vi "FindMessageSet.vi"(11 "ConcreteActor.lvclass":variant) -> (3 "MessageSet":T1)   [LabVIEW 2020, in "jettl.lvlib"]
uses:
  jettl.lvlib
  Message/Message.lvclass
  MessageSet.ctl
  <vilib>/Utility/Data Type/NI_Data Type.lvlib
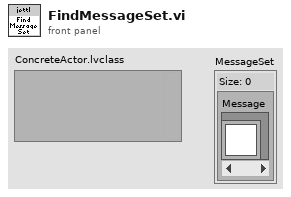
[diagram p1: front panel]
types:
  T1 = typedef "jettl.lvlib/MessageSet.ctl" = set{refnum<class "Message.lvclass">}
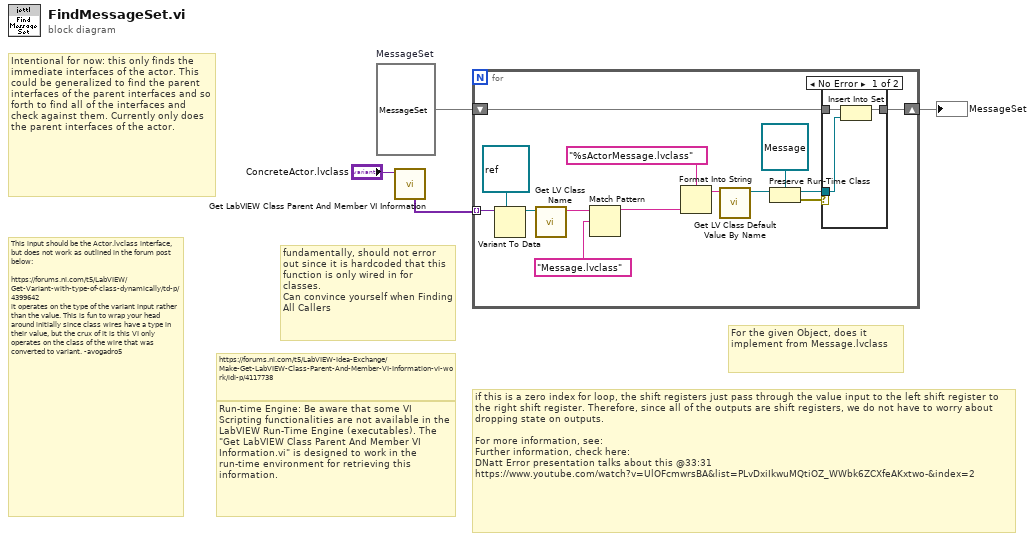
[diagram p0: block diagram]
diagram:
  w4 = T1 {}  # MessageSet
  # "fundamentally, should not error out since it is hardcoded that this function is only wired in for classes.\nCan convince yourself when Finding All Callers"
  # "if this is a zero index for loop, the shift registers just pass through the value input to the left shift register to the right shift register. Therefore, since all of the outputs are shift registers, we do not have to worry about dropping state on outputs.\n\nFor more information, see:\nFurther information, check here:\nDNatt Error presentation talks about this @33:31\nhttps://www.youtube.com/watch?v=UlOFcmwrsBA&list=PLvDxiIkwuMQtiOZ_WWbk6ZCXfeAKxtwo-&index=2"
  # "For the given Object, does it implement from Message.lvclass"
  # "This input should be the Actor.lvclass interface, but does not work as outlined in the forum post below:\n\nhttps://forums.ni.com/t5/LabVIEW/Get-Variant-with-type-of-class-dynamically/td-p/4399642\nit operates on the type of the variant input rather than the value. This is fun to wrap your head around initially since class wires have a type in their value, but the crux of it is this VI only operates on the class of the wire that was converted to variant. -avogadro5"
  # "Intentional for now: this only finds the immediate interfaces of the actor. This could be generalized to find the parent interfaces of the parent interfaces and so forth to find all of the interfaces and check against them. Currently only does the parent interfaces of the actor."
  # "Run-time Engine: Be aware that some VI Scripting functionalities are not available in the LabVIEW Run-Time Engine (executables). The \"Get LabVIEW Class Parent And Member VI Information.vi\" is designed to work in the run-time environment for retrieving this information."
  # "https://forums.ni.com/t5/LabVIEW-Idea-Exchange/Make-Get-LabVIEW-Class-Parent-And-Member-VI-Information-vi-work/idi-p/4117738"
  n1 = call <vilib>:"Get LabVIEW Class Parent And Member VI Information.vi"("variant"="ConcreteActor.lvclass") -> ("parent interfaces"=w1:variant[])  [unwired: 7 in, 3 out]
  n2 = for {
    tunnel: w1 -> [w17] mode=indexing
    shift-right: [w13] -> w3
    shift-left: w4 -> [w14]
    n3 = Variant To Data(type=refnum<class> refnum ("LabVIEW Object"), Variant=w17) -> (data=w16:refnum<class>)  [unwired: 1 in, 1 out]
    n4 = call <vilib>:"Get LV Class Name.vi"("object"=w16) -> ("class name"=w7:string)  [unwired: 9 in, 1 out]
    n5 = Match Pattern(string=w7, regular expression="Message.lvclass" ("string")) -> (before substring=w6:string)  [unwired: 1 in, 3 out]
    n6 = Format Into String(format string="%sActorMessage.lvclass", w6) -> (resulting string=w5:string)  [unwired: 2 in, 1 out]
    n7 = call <vilib>:"Get LV Class Default Value By Name.vi"("class name"=w5) -> ("object"=w15:refnum<class>)  [unwired: 9 in, 1 out]
    n8 = Preserve Run-Time Class(object in=w15, 2:refnum<class "Message.lvclass"> refnum ("Msg")) -> (object out=w10:refnum<class "Message.lvclass">, error out=w8:errorcluster)  [unwired: 1 in]
    n9 = case shown="No Error" w8 {
      tunnel: w14 -> [w21 w22]
      tunnel: [w20 w22] -> w13
      tunnel: w10 -> [w19 _]
      frame No Error {
        n10 = Insert Into Set(10:w19, 11:w21) -> (3:w20:T1)  [unwired: 1 out]
      }
      frame Error {
      }
    }
  }
  "MessageSet" <- w3
